vi "PWM.vi"() -> ()   [LabVIEW 2018]
uses:
  <vilib>/rvi/Emulation/niFpgaGetClockAttributes.vi
  <vilib>/rvi/Emulation/niFpgaSctlEmulationGetInTimedLoop.vi
  <vilib>/rvi/Emulation/niFpgaEmulationReportErrorSimple.vi
  <vilib>/rvi/eio/common/nirviEmuTemplateMethod_errors.vi
  <vilib>/rvi/Emulation/niFpgaCriticalErrorInLSC.vi
  <vilib>/eio/EIONode/EIONode.xnode
panel:
  in  "servo pwm":u32(slide) caption="Tick Count(uSec)" scale=0.0..80.0
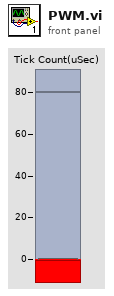
[diagram p1: front panel]
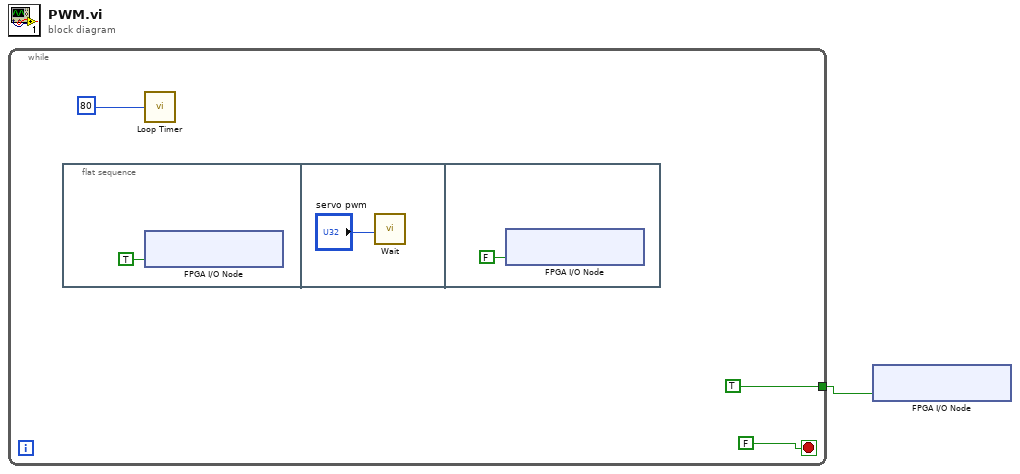
[diagram p0: block diagram]
diagram:
  n1 = while {
    tunnel: [TRUE] -> w1
    stop <- FALSE stop-if-true
    n2 = flat-sequence {
      frame #0 {
        n3 = xnode "FPGA I/O Node"("ConnectorA/DIO9"=TRUE ("ConnectorA/DIO0")) -> ()  [unwired: 1 in, 1 out]
      }
      frame #1 {
        n4 = call "Wait"("Count(uSec)"="servo pwm") -> ()  [unwired: 1 out]
      }
      frame #2 {
        n5 = xnode "FPGA I/O Node"("ConnectorA/DIO9"=FALSE ("ConnectorA/DIO0")) -> ()  [unwired: 1 in, 1 out]
      }
    }
    n6 = call "Loop Timer"("Count(uSec)"=i16 80) -> ()  [unwired: 1 out]
  }
  n7 = xnode "FPGA I/O Node"("ConnectorA/DIO9"=w1) -> ()  [unwired: 1 in, 1 out]
